vi "SaveTrendPoints.vi"(8 "error in (no error)":errorcluster, 9 "data":T1, 10 "data event in":T6, 11 "config in":T5) -> (0 "error out":errorcluster, 2 "data event out":T6)   [LabVIEW 2017, in "IrDataEventCreator.lvlib"]
uses:
  <vilib>/addons/InsightCM/Devices/Shared/Ir/IrDataEventCreator/IrDataEventCreator.lvlib
  <vilib>/addons/InsightCM/Devices/Shared/Common/DataEvent/controls/Event.ctl
  <vilib>/addons/InsightCM/MessageBus/Base/controls/DataEvent.ctl
  <vilib>/addons/InsightCM/MessageBus/Base/controls/KeyValuePair.ctl
  <vilib>/addons/InsightCM/Devices/Shared/Common/DataEvent/controls/DataSet.ctl
  <vilib>/addons/InsightCM/MessageBus/Base/controls/DataSetMetadata.ctl
  <vilib>/addons/InsightCM/MessageBus/Base/controls/TrendPoint.ctl
  <vilib>/addons/InsightCM/MessageBus/Base/controls/TrendAlarmUpdate.ctl
  <vilib>/addons/InsightCM/MessageBus/Base/controls/TrendAlarmTransition.ctl
  <vilib>/addons/InsightCM/Devices/Shared/Ir/IrDataEventCreator/controls/config.ctl
  <vilib>/addons/InsightCM/Devices/Shared/Common/DataFlow/controls/Data.ctl
  <vilib>/addons/InsightCM/Utilities/DataAccessors/controls/wfmSGL_DVR.ctl
  <vilib>/addons/PointValueMap/controls/PointMap.ctl
  <vilib>/addons/InsightCM/Devices/Shared/Common/DataFlow/controls/Type.ctl
  <vilib>/addons/InsightCM/Devices/Shared/Ir/IrDataEventCreator/controls/Registry.ctl
  <vilib>/addons/InsightCM/Devices/Shared/Ir/IrDataEventCreator/controls/Registry_Image.ctl
  <vilib>/addons/InsightCM/Devices/Shared/Common/DataEventCreator/controls/Registry_Trend.ctl
  <vilib>/addons/PointValueMap/subVIs/Point_Read_double.vi
  <vilib>/addons/PointValueMap/PointValueMap.lvlib
  <vilib>/addons/InsightCM/Devices/Shared/Common/DataEventCreator/DataEventCreator.lvlib
  <vilib>/addons/InsightCM/Devices/Shared/Common/DataEvent/DataEvent.lvlib
  <vilib>/addons/InsightCM/Devices/Shared/Common/DataFlow/DataFlow.lvlib
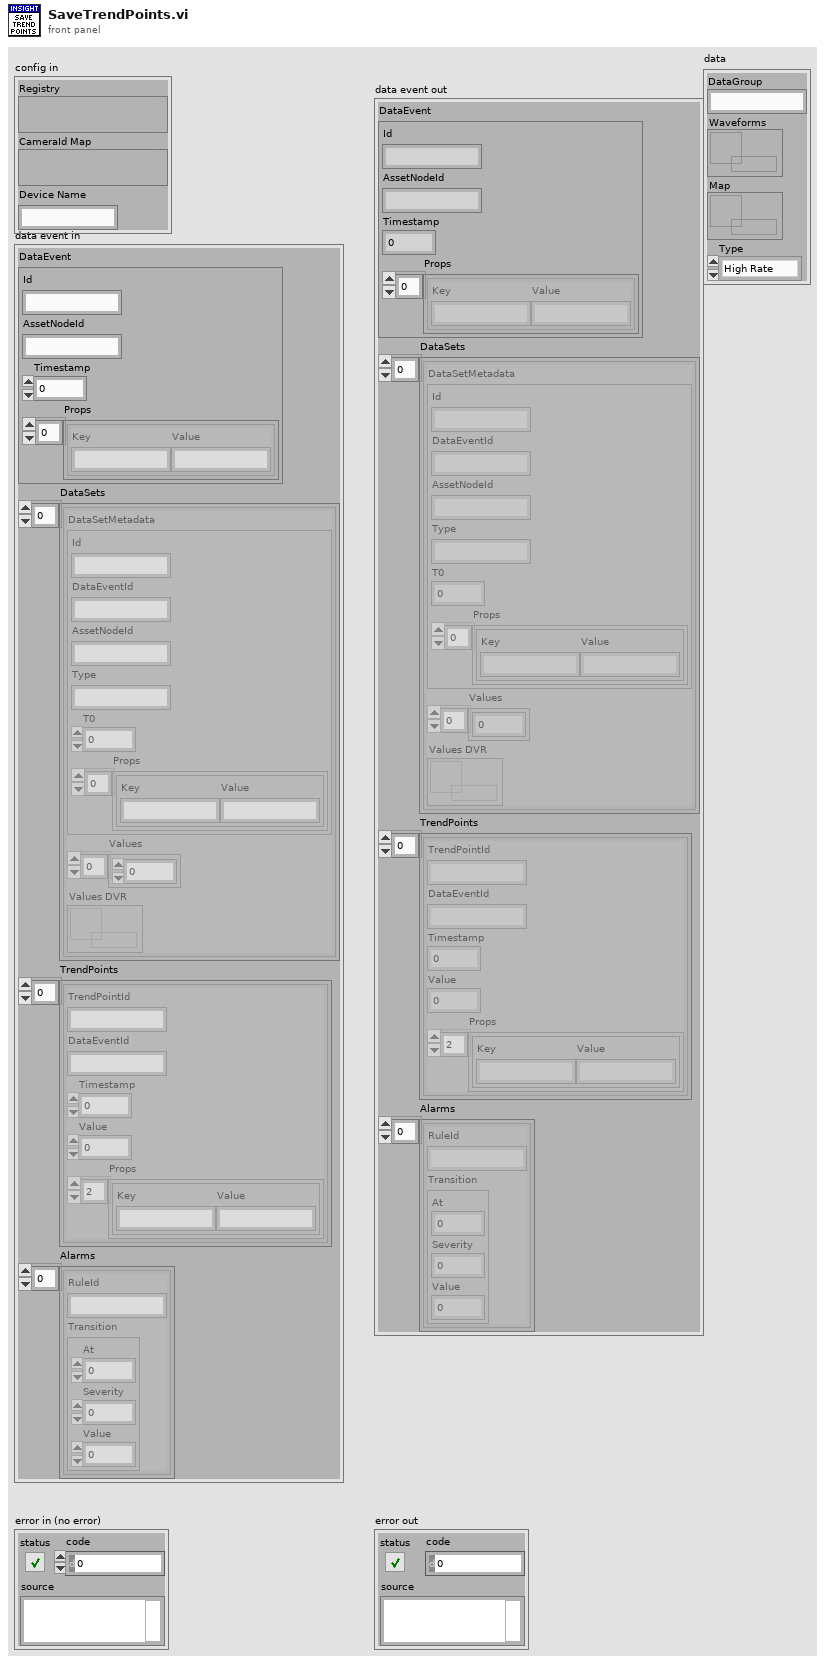
[diagram p1: front panel]
types:
  T1 = typedef "DataFlow.lvlib/Data.ctl" = cluster{"DataGroup":string, "Waveforms":T2, "Map":T3, "Type":T4}
  T2 = typedef "wfmSGL_DVR.ctl" = refnum<data-value>
  T3 = typedef "PointValueMap.lvlib/PointMap.ctl" = refnum<data-value>
  T4 = typedef "DataFlow.lvlib/Type.ctl" = enum16{"High Rate", "Low Rate", "Burst Mode"}
  T5 = typedef "IrDataEventCreator.lvlib/config.ctl" = cluster{"Registry":variant, "CameraId Map":variant, "Device Name":string}
  T6 = typedef "DataEvent.lvlib/Event.ctl" = cluster{"DataEvent":T7, "DataSets":T9[], "TrendPoints":T11[], "Alarms":T12[]}
  T7 = typedef "DataEvent.ctl" = cluster{"Id":string, "AssetNodeId":string, "Timestamp":i64, "Props":T8[]}
  T8 = typedef "KeyValuePair.ctl" = cluster{"Key":string, "Value":string}
  T9 = typedef "DataEvent.lvlib/DataSet.ctl" = cluster{"DataSetMetadata":T10, "Values":sgl[], "Values DVR":refnum<data-value>}
  T10 = typedef "DataSetMetadata.ctl" = cluster{"Id":string, "DataEventId":string, "AssetNodeId":string, "Type":string, "T0":i64, "Props":T8[]}
  T11 = typedef "TrendPoint.ctl" = cluster{"TrendPointId":string, "DataEventId":string, "Timestamp":i64, "Value":dbl, "Props":T8[]}
  T12 = typedef "TrendAlarmUpdate.ctl" = cluster{"RuleId":string, "Transition":T13}
  T13 = typedef "TrendAlarmTransition.ctl" = cluster{"At":i64, "Severity":i32, "Value":dbl}
  T14 = typedef "IrDataEventCreator.lvlib/Registry.ctl" = cluster{"Image":T15, "Trend Points":T16[]}
  T15 = typedef "IrDataEventCreator.lvlib/Registry_Image.ctl" = cluster{"Properties":T8[]}
  T16 = typedef "DataEventCreator.lvlib/Registry_Trend.ctl" = cluster{"TrendPointId":string, "DataSetName":string, "HighRate":bool, "Always Send":bool}
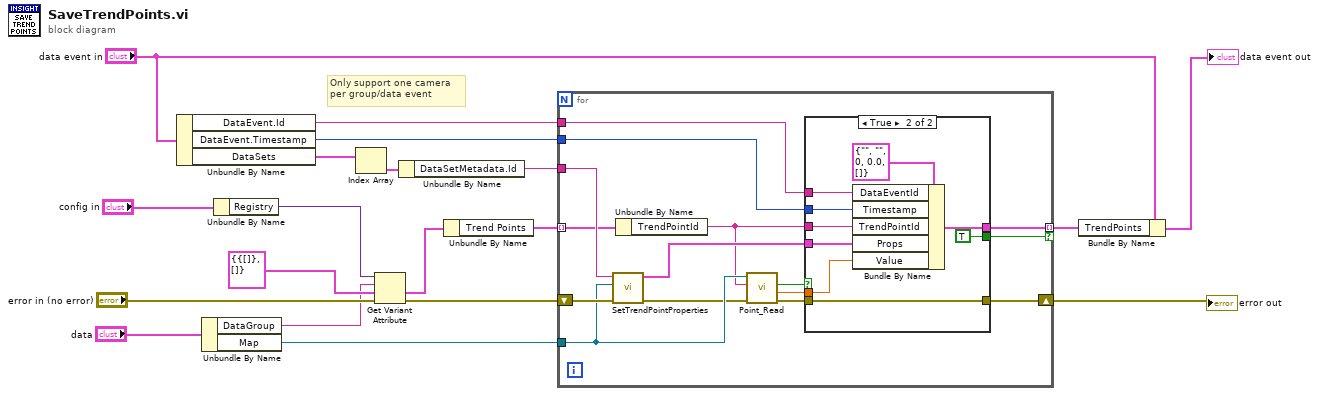
[diagram p0: block diagram]
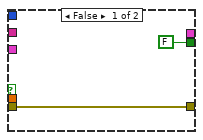
[diagram p2: hidden frame]
diagram:
  # "Only support one camera\nper group/data event"
  n1 = Unbundle By Name("data event in") -> ("DataEvent.Id"=w2:string, "DataEvent.Timestamp"=w4:i64, "DataSets"=w7:T9[])
  n2 = Unbundle By Name("data") -> ("DataGroup"=w13:string, "Map"=w9:T3)
  n3 = Unbundle By Name("config in") -> ("Registry"=w16:variant)
  n4 = Index Array(array=w7) -> (element=w6:T9)  [unwired: 1 in]
  n5 = Get Variant Attribute(Variant=w16, name=w13, default value (empty Variant)=T14 {"Image"={"Properties"=[]}, "Trend Points"=[]} ("Registry"), error in="error in (no error)") -> (value=w12:T14, error out=w10:errorcluster)  [unwired: 2 out]
  n6 = Unbundle By Name(w6) -> ("DataSetMetadata.Id"=w5:string)
  n7 = Unbundle By Name(w12) -> ("Trend Points"=w11:T16[])
  n8 = for {
    tunnel: w11 -> [w30] mode=indexing
    shift-right: [w22] -> w1
    shift-left: w10 -> [w34]
    tunnel: w9 -> [w27]
    tunnel: w5 -> [w33]
    tunnel: w4 -> [w32]
    tunnel: [w31] -> w3 mode=indexing if=w20
    tunnel: w2 -> [w28]
    n9 = call <vilib>:"SetTrendPointProperties.vi"("error in (no error)"=w34, "map"=w27, "data set id"=w33) -> ("error out"=w26:errorcluster, "properties"=w29:T8[])  [unwired: 7 in]
    n10 = Unbundle By Name(w30) -> ("TrendPointId"=w25:string)
    n11 = call-poly <vilib>:"Point_Read.vi"("Error In"=w26, "Tag"=w25, "Map"=w27) -> ("Error Out"=w21:errorcluster, "Value"=w24:dbl, "Found?"=w23:bool)  [unwired: 3 in, 3 out]
    n12 = case shown="True" w23 {
      tunnel: w32 -> [_ w44]
      tunnel: [_ w43] -> w31
      tunnel: w29 -> [_ w42]
      tunnel: w28 -> [_ w41]
      tunnel: w25 -> [_ w40]
      tunnel: w24 -> [_ w39]
      tunnel: [w35 w38] -> w22
      tunnel: w21 -> [w35 w38]
      tunnel: [FALSE TRUE] -> w20
      frame False {
      }
      frame True {
        n13 = Bundle By Name(cluster=T11 {"TrendPointId"="", "DataEventId"="", "Timestamp"=0, "Value"=0.0, "Props"=[]} ("TrendPoint"), "DataEventId"=w41, "Timestamp"=w44, "TrendPointId"=w40, "Props"=w42, "Value"=w39) -> (w43:T11)
      }
    }
  }
  "error out" <- w1
  n14 = Bundle By Name(cluster="data event in", "TrendPoints"=w3) -> (→"data event out":T6)
